vi "Read Field.vi"(4 "Properties":T2 {"Common"."Address" format="%x"}, 6 "LinkData":T15, 8 "Error In":errorcluster, 10 "Link":T16, 11 "WorkspaceManager":T1) -> (0 "Error Out":errorcluster, 1 "NewVal":bool, 2 "Table":cluster{"X":sgl[], "Y":sgl[], "Z":sgl[][]}, 3 "WorkspaceManager out":T1)   [LabVIEW 2011]
uses:
  Controls/ECUMC Item.ctl
  Controls/LinkData.ctl
  <vilib>/ECUMC/NIVS/Support Files.llb/Item Properties.ctl
  <vilib>/ECUMC/NIVS/Support Files.llb/Address Property.ctl
  <vilib>/ECUMC/NIVS/Support Files.llb/Extension Property.ctl
  <vilib>/ECUMC/NIVS/Support Files.llb/Data Type Property.ctl
  <vilib>/ECUMC/NIVS/Support Files.llb/Byte Order Property.ctl
  <vilib>/ECUMC/NIVS/Support Files.llb/Maximum Property.ctl
  <vilib>/ECUMC/NIVS/Support Files.llb/Minimum Property.ctl
  <vilib>/ECUMC/NIVS/Support Files.llb/Read Only Property.ctl
  <vilib>/ECUMC/NIVS/Support Files.llb/Unit Property.ctl
  <vilib>/ECUMC/NIVS/Support Files.llb/Comment Property.ctl
  <vilib>/ECUMC/NIVS/Support Files.llb/X Dimension Property.ctl
  <vilib>/ECUMC/NIVS/Support Files.llb/Y Dimension Property.ctl
  <vilib>/ECUMC/NIVS/Support Files.llb/Is Virtual Property.ctl
  <vilib>/NI Veristand/Execution/Workspace/WorkspaceAPI.ctl
  NationalInstruments.VeriStand.ClientAPI
  <vilib>/ECUMC/NIVS/Support Files.llb/Get Single Char Data (TCP).vi
  <vilib>/NI Veristand/Execution/Workspace/NI VeriStand - Get Multiple Channel Values.vi
  <vilib>/ECUMC/NIVS/XCPCCP Add-On Execution API.lvlib
  <vilib>/NI Veristand/Execution/Workspace/NI_VS Workspace ExecutionAPI.lvlib
  <vilib>/ECUMC/NIVS/Support Files.llb/XCP and CCP Master Custom Device.lvlib
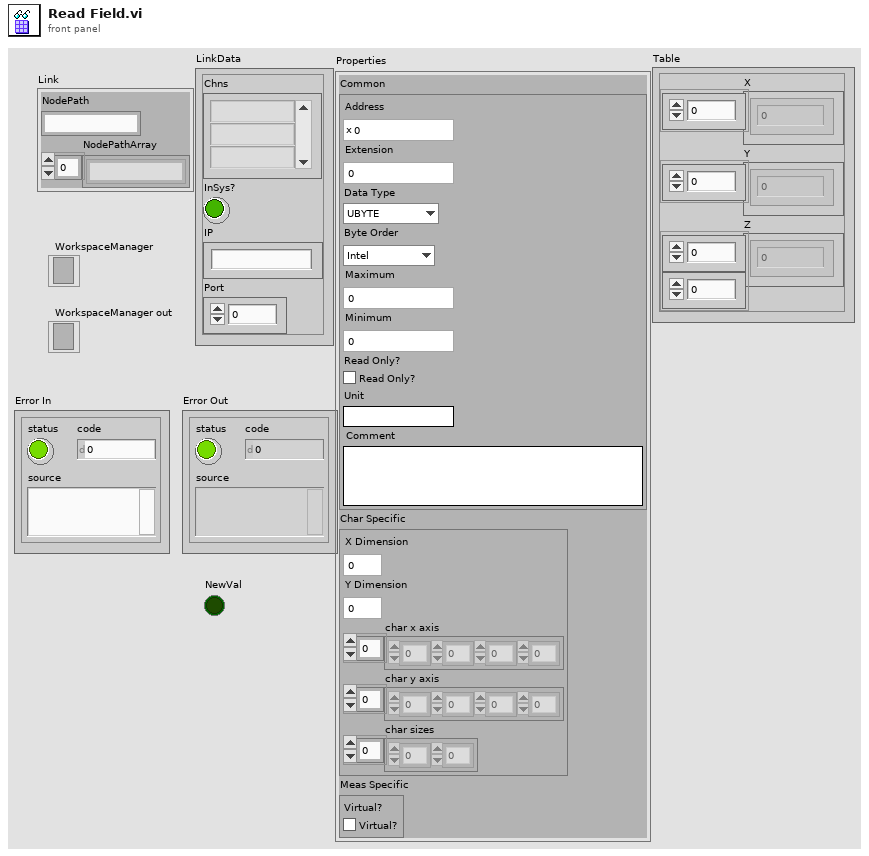
[diagram p1: front panel]
types:
  T1 = typedef "NI_VS Workspace ExecutionAPI.lvlib/WorkspaceAPI.ctl" = refnum<k24>
  T2 = typedef "XCP and CCP Master Custom Device.lvlib/Item Properties.ctl" = cluster{"Common":cluster{"Address":T3, "Extension":T4, "Data Type":T5, "Byte Order":T6, "Maximum":T7, "Minimum":T8, "Read Only?":T9, "Unit":T10, "Comment":T11}, "Char Specific":cluster{"X Dimension":T12, "Y Dimension":T13, "char x axis":dbl[], "char y axis":dbl[], "char sizes":u32[]}, "Meas Specific":cluster{"Virtual?":T14}}
  T3 = typedef "XCP and CCP Master Custom Device.lvlib/Address Property.ctl" = u32
  T4 = typedef "XCP and CCP Master Custom Device.lvlib/Extension Property.ctl" = u8
  T5 = typedef "XCP and CCP Master Custom Device.lvlib/Data Type Property.ctl" = enum16{"UBYTE", "SBYTE", "UWORD", "SWORD", "ULONG", "SLONG", "FLOAT32_IEEE", "FLOAT64_IEEE"}
  T6 = typedef "XCP and CCP Master Custom Device.lvlib/Byte Order Property.ctl" = enum16{"Intel", "Motorola"}
  T7 = typedef "XCP and CCP Master Custom Device.lvlib/Maximum Property.ctl" = dbl
  T8 = typedef "XCP and CCP Master Custom Device.lvlib/Minimum Property.ctl" = dbl
  T9 = typedef "XCP and CCP Master Custom Device.lvlib/Read Only Property.ctl" = bool
  T10 = typedef "XCP and CCP Master Custom Device.lvlib/Unit Property.ctl" = string
  T11 = typedef "XCP and CCP Master Custom Device.lvlib/Comment Property.ctl" = string
  T12 = typedef "XCP and CCP Master Custom Device.lvlib/X Dimension Property.ctl" = u32
  T13 = typedef "XCP and CCP Master Custom Device.lvlib/Y Dimension Property.ctl" = u32
  T14 = typedef "XCP and CCP Master Custom Device.lvlib/Is Virtual Property.ctl" = bool
  T15 = typedef "LinkData.ctl" = cluster{"Chns":string[], "InSys?":bool, "IP":string, "Port":u16}
  T16 = typedef "ECUMC Item.ctl" = cluster{"NodePath":string, "NodePathArray":string[]}
  T17 = typedef "XCP and CCP Master Custom Device.lvlib/Char Data (TCP).ctl" = cluster{"1d":dbl[], "2d":dbl[][], "Single":dbl, "Size":T18}
  T18 = typedef "XCP and CCP Master Custom Device.lvlib/Char Size for TCP.ctl" = enum16{"Single", "1d", "2d"}
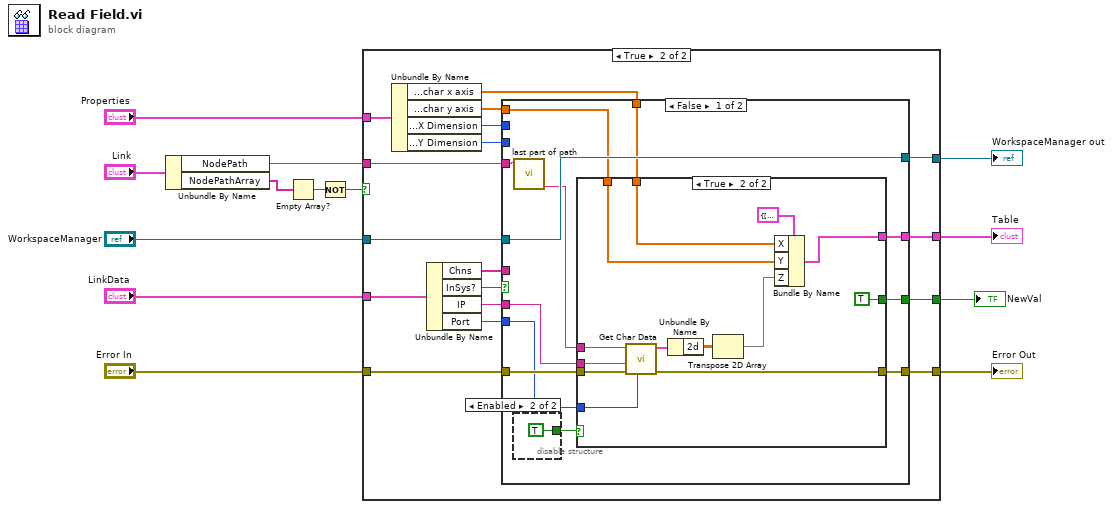
[diagram p0: block diagram]
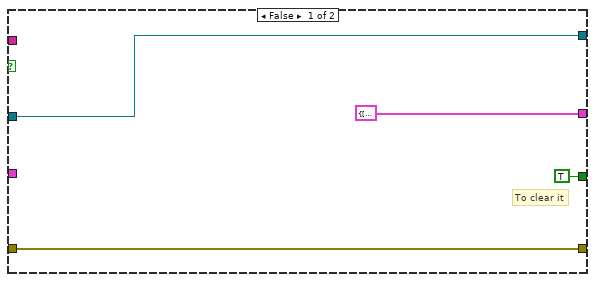
[diagram p2: hidden frame]
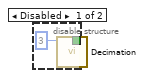
[diagram p3: hidden frame]
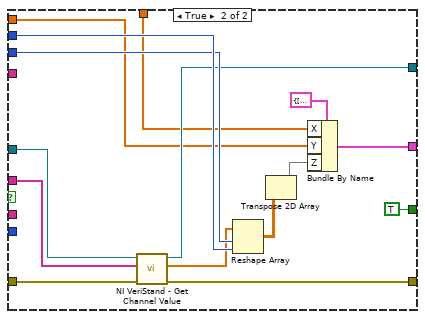
[diagram p5: hidden frame]
diagram:
  n1 = Unbundle By Name("Link") -> ("NodePath"=w10:string, "NodePathArray"=w5:string[])
  n2 = Empty Array?(array=w5) -> (empty?=w3:bool)
  n3 = Not(x=w3) -> (.not. x?=w2:bool)
  n4 = case shown="True" w2 {
    tunnel: "LinkData" -> [_ w34]
    tunnel: "Error In" -> [w17 w31]
    tunnel: w10 -> [_ w19]
    tunnel: "Properties" -> [_ w23]
    tunnel: [cluster{"X":sgl[], "Y":sgl[], "Z":sgl[][]} {"X"=[], "Y"=[], "Z"=[]} ("TBL2D") w20] -> w8
    tunnel: "WorkspaceManager" -> [w16 w26]
    tunnel: [w17 w25] -> w6
    tunnel: [w16 w24] -> w4
    tunnel: [TRUE w18] -> w1
    frame False {
      # "To clear it"
    }
    frame True {
      n5 = Unbundle By Name(w23) -> ("Char Specific.char x axis"=w21:dbl[], "Char Specific.char y axis"=w22:dbl[], "Char Specific.X Dimension"=w28:T12, "Char Specific.Y Dimension"=w27:T13)
      n6 = Unbundle By Name(w34) -> ("Chns"=w32:string[], "InSys?"=w33:bool, "IP"=w30:string, "Port"=w29:u16)
      n7 = case shown="False" w33 {
        tunnel: w32 -> [_ w78]
        tunnel: w26 -> [w42 w77]
        tunnel: w31 -> [w46 w76]
        tunnel: [w45 w75] -> w25
        tunnel: w30 -> [w44 _]
        tunnel: w29 -> [w43 _]
        tunnel: w28 -> [_ w74]
        tunnel: w27 -> [_ w73]
        tunnel: [w42 w71] -> w24
        tunnel: w22 -> [w40 w68]
        tunnel: w21 -> [w39 w69]
        tunnel: [w38 w65] -> w20
        tunnel: w19 -> [w37 _]
        tunnel: [w35 TRUE] -> w18
        frame False {
          n8 = call "last part of path.vi"("String"=w37) -> ("Last Part"=w36:string)  [unwired: 10 in]
          n9 = disable-structure shown="Enabled" {
            disable-tunnel: [w47 TRUE ("Trigger")] -> w41
            frame Disabled {
              n10 = call "Decimation.vi"("Decimation Factor"=3) -> ("Trigger"=w47:bool)  [unwired: 10 in]
            }
            frame Enabled {
            }
          }
          n11 = case shown="True" w41 {
            tunnel: w46 -> [w50 w63]
            tunnel: [w50 w62] -> w45
            tunnel: w44 -> [_ w61]
            tunnel: w43 -> [_ w60]
            tunnel: w36 -> [_ w58]
            tunnel: w40 -> [_ w56]
            tunnel: w39 -> [_ w54]
            tunnel: [_ w52] -> w38
            tunnel: [_ TRUE] -> w35
            frame False {
            }
            frame True {
              n12 = call-poly <vilib>:"Get Char Data.vi"("Port"=w60, "error in (no error)"=w63, "IP or DNS Name"=w61, "Characteristic"=w58) -> ("error out"=w62:errorcluster, "Characteristic Data"=w59:T17)  [unwired: 6 in]
              n13 = Unbundle By Name(w59) -> ("2d"=w55:dbl[][])
              n14 = Transpose 2D Array(2D array=w55) -> (transposed array=w53:dbl[][])
              n15 = Bundle By Name(cluster=cluster{"X":sgl[], "Y":sgl[], "Z":sgl[][]} {"X"=[], "Y"=[], "Z"=[]} ("TBL2D"), "X"=w54, "Y"=w56, "Z"=w53) -> (w52:cluster{"X":sgl[], "Y":sgl[], "Z":sgl[][]})
            }
          }
        }
        frame True {
          n16 = call-poly <vilib>:"NI VeriStand - Get Channel Value.vi"("error in (no error)"=w76, "Channels"=w78, "WorkspaceManager in"=w77) -> ("error out"=w75:errorcluster, "Values"=w72:dbl[], "WorkspaceManager out"=w71:T1)  [unwired: 6 in]
          n17 = Reshape Array(w72, w73, w74) -> (w67:dbl[][])
          n18 = Transpose 2D Array(2D array=w67) -> (transposed array=w66:dbl[][])
          n19 = Bundle By Name(cluster=cluster{"X":sgl[], "Y":sgl[], "Z":sgl[][]} {"X"=[], "Y"=[], "Z"=[]} ("TBL2D"), "X"=w69, "Y"=w68, "Z"=w66) -> (w65:cluster{"X":sgl[], "Y":sgl[], "Z":sgl[][]})
        }
      }
    }
  }
  "Error Out" <- w6
  "WorkspaceManager out" <- w4
  "Table" <- w8
  "NewVal" <- w1
